vi "Periodic Tasks.vi"(8 "error in":errorcluster) -> ()   [LabVIEW 2012]
doc: "This VI runs in parallel to other tasks. It can contain as many user-defined periodic loops as you need. These can carry out PID or other sorts of timed response."
uses:
  <vilib>/Rock Robotics/SystemInterfaces/Utilities/FPGA_UtilitiesLED Source.ctl
  <vilib>/Rock Robotics/SystemInterfaces/Utilities/FPGA_UtilitiesLED State.ctl
  Robot Global Data.vi
  BotStatus.vi
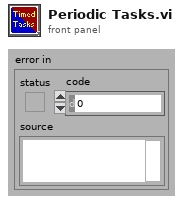
[diagram p1: front panel]
types:
  T1 = typedef "FPGA_UtilitiesLED State.ctl" = enum16{"Off", "On", "Toggle"}
  T2 = typedef "FPGA_UtilitiesLED Source.ctl" = enum16{"User LED", "FPGA LED"}
  T3 = typedef "WPI_ServoDeviceRef.ctl" = cluster{"DeviceStatus":errorcluster, "Digital Module":T4, "PWM Channel":T5, "DeadBand":T6}
  T4 = typedef "FPGA_TypedefDigitalModule.ctl" = enum16{"Digital Module 1", "Digital Module 2"}
  T5 = typedef "FPGA_DIOPWMChannel.ctl" = enum8{"PWM 1", "PWM 2", "PWM 3", "PWM 4", "PWM 5", "PWM 6", "PWM 7", "PWM 8", "PWM 9", "PWM 10", "Invalid"}
  T6 = typedef "WPI_PWMDeadband.ctl" = cluster{"Name":string, "maxPositivePwm":i32, "minPositivePwm":i32, "centerPwm":i32, "maxNegativePwm":i32, "minNegativePwm":i32, "angularRange":u16}
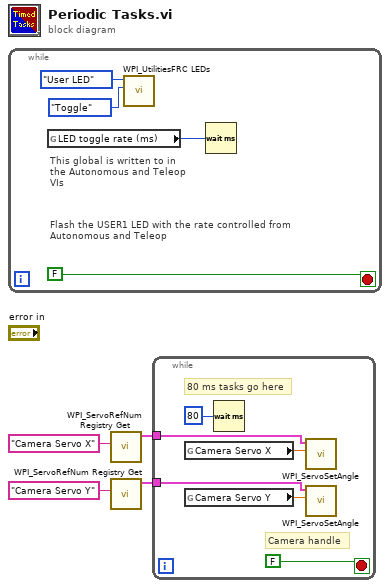
[diagram p0: block diagram]
diagram:
  n1 = while {
    stop <- FALSE stop-if-true
    # "This global is written to in the Autonomous and Teleop VIs"
    # "Flash the USER1 LED with the rate controlled from Autonomous and Teleop"
    n2 = global read "Robot Global Data.vi" "LED toggle rate (ms)"() -> (w5:u32)
    n3 = call <vilib>:"WPI_UtilitiesFRC LEDs.vi"("State"=FPGA_UtilitiesLED_State."Toggle", "LED Type"=FPGA_UtilitiesLED_Source."User LED") -> ()  [unwired: 1 in, 9 out]
    n4 = Wait (ms)(milliseconds to wait=w5) -> ()  [unwired: 1 out]
  }
  n5 = call <vilib>:"WPI_ServoRefNum Registry Get.vi"("refnum name"="Camera Servo X") -> ("ServoDeviceRef"=w3:T3)  [unwired: 9 in, 1 out]
  n6 = call <vilib>:"WPI_ServoRefNum Registry Get.vi"("refnum name"="Camera Servo Y") -> ("ServoDeviceRef"=w1:T3)  [unwired: 9 in, 1 out]
  n7 = while {
    tunnel: w3 -> [w12]
    tunnel: w1 -> [w11]
    stop <- FALSE stop-if-true
    # "Camera handle"
    # "80 ms tasks go here"
    n8 = global read "BotStatus.vi" "Camera Servo X"() -> (w10:dbl)
    n9 = global read "BotStatus.vi" "Camera Servo Y"() -> (w9:dbl)
    n10 = Wait (ms)(milliseconds to wait=u32 80) -> ()  [unwired: 1 out]
    n11 = call <vilib>:"WPI_ServoSetAngle.vi"("Angle"=w10, "ServoDeviceRef"=w12) -> ()  [unwired: 8 in, 2 out]
    n12 = call <vilib>:"WPI_ServoSetAngle.vi"("Angle"=w9, "ServoDeviceRef"=w11) -> ()  [unwired: 8 in, 2 out]
  }
